vi "FRIC_navX_Util_DecodeProtocol_UInt16.vi"(5 "Device Number":T1, 8 "length":i32=2, 9 "Device Register":T2=18 items=["WHOAMI"=0, "HW_REV"=1, "FW_VER_MAJOR"=2, "FW_VER_MINOR"=3, "UPDATE_RATE_HZ"=4, "ACCEL_FSR_G"=5, "GYRO_FSR_DPS"=6, "OP_STATUS"=8, "CAL_STATUS"=9, "SELFTEST_STATUS"=10, "CAPABILITY_FLAGS_L"=11, "CAPABILITY_FLAGS_H"=12, "SENSOR_STATUS"=16, "TIMESTAMP"=18, "YAW"=22, "ROLL"=24, "PITCH"=26, "HEADING"=28, "FUSED_HEADING"=30, "ALTITUDE_I"=32, "ALTITUDE_D"=34, "LINERA_ACC_X"=36, "LINERA_ACC_Y"=38, "LINERA_ACC_Z"=40, "QUAT_W"=42, "QUAT_X"=44, "QUAT_Y"=46, "QUAT_Z"=48, "MPU_TEMP_C"=50, "GYRO_X"=52, "GYRO_Y"=54, "GYRO_Z"=56, "ACC_X"=58, "ACC_Y"=60, "ACC_Z"=62, "MAG_X"=64, "MAG_Y"=66, "MAG_Z"=68, "PRESSURE_I"=70, "PRESSURE_D"=72, "PRESSURE_TEMP"=74, "YAW_OFFSET"=76, "QUAT_OFFSET_W"=78, "QUAT_OFFSET_X"=80, "QUAT_OFFSET_Y"=82, "QUAT_OFFSET_Z"=84, "INTEGRATION_CONTROL"=86, "VELOCITY_X"=88, "VELOCITY_Y"=92, "VELOCITY_Z"=96, "DISPLACMENT_X"=100, "DISPLACMENT_Y"=104, "DISPLACEMENT_Z"=108]) -> (3 "Value":u16)   [LabVIEW 2019]
uses:
  <vilib>/Rock Robotics/WPI/ThirdParty/Sensors/navX/_TypeDefs/Z900_navX_DeviceRegisters.ctl
  <vilib>/Rock Robotics/WPI/ThirdParty/Sensors/navX/_TypeDefs/FRIC_navX_DeviceNumbersTypeDef.ctl
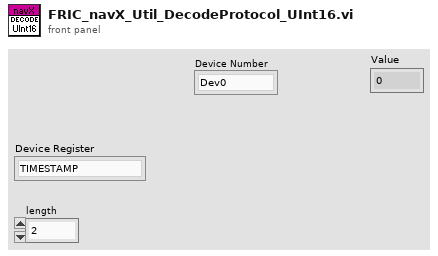
[diagram p1: front panel]
types:
  T1 = typedef "FRIC_navX_DeviceNumbersTypeDef.ctl" = enum16{"Dev0", "Dev1", "Dev2", "Dev3"}
  T2 = typedef "Z900_navX_DeviceRegisters.ctl" = u8
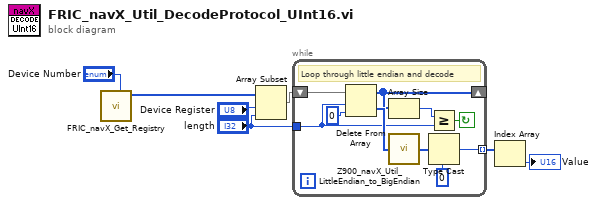
[diagram p0: block diagram]
diagram:
  n1 = call <vilib>:"FRIC_navX_Get_Registry.vi"("Device Number"="Device Number") -> ("Registry (out)"=w2:u8[])  [unwired: 9 in, 1 out]
  n2 = Array Subset(array=w2, index="Device Register", length="length") -> (w6:u8[])
  n3 = while {
    shift-right: [w11] -> _
    shift-left: w6 -> [w17]
    tunnel: [w12] -> w4 mode=indexing
    tunnel: "length" -> [w8]
    stop <- w9 continue-if-true
    # "Loop through little endian and decode"
    n4 = Delete From Array(array=w17, length=w8, index=0) -> (deleted portion=w13:u8[], array with subset deleted=w11:u8[])
    n5 = Array Size(array=w11) -> (size(s)=w10:i32)
    n6 = call <vilib>:"Z900_navX_Util_LittleEndian_to_BigEndian.vi"("Little Endian"=w13) -> ("Big Endian"=w15:u8[])
    n7 = Greater Or Equal?(x=w10, y=w8) -> (x >= y?=w9:bool)
    n8 = Type Cast(type=u16 0, x=w15) -> (*(type *) &x=w12:u16)
  }
  n9 = Index Array(array=w4) -> (element=→"Value":u16)  [unwired: 1 in]
